vi "Double to RGB Image.vi"(8 "error in (no error)":errorcluster, 9 "minimum":sgl, 10 "maximum":sgl, 11 "Image Reference In":T1) -> (0 "error out":errorcluster, 3 "Image Reference Out":T1)   [LabVIEW 2019]
doc: "This VI converts a double image to a U8 image by converting the pixels from values in a particular range to 0-255 and adding them to a new image."
uses:
  <vilib>/vision/Image Controls.llb/IMAQ Image.ctl
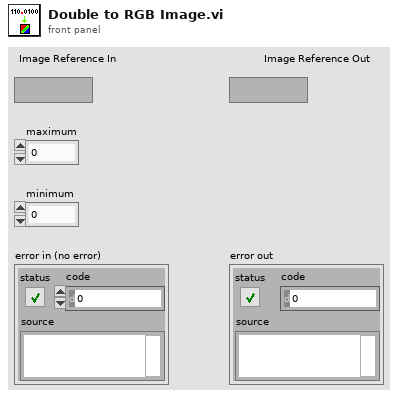
[diagram p1: front panel]
types:
  T1 = typedef "IMAQ Image.ctl" = refnum<image>
  T2 = typedef "Image Type" = u32
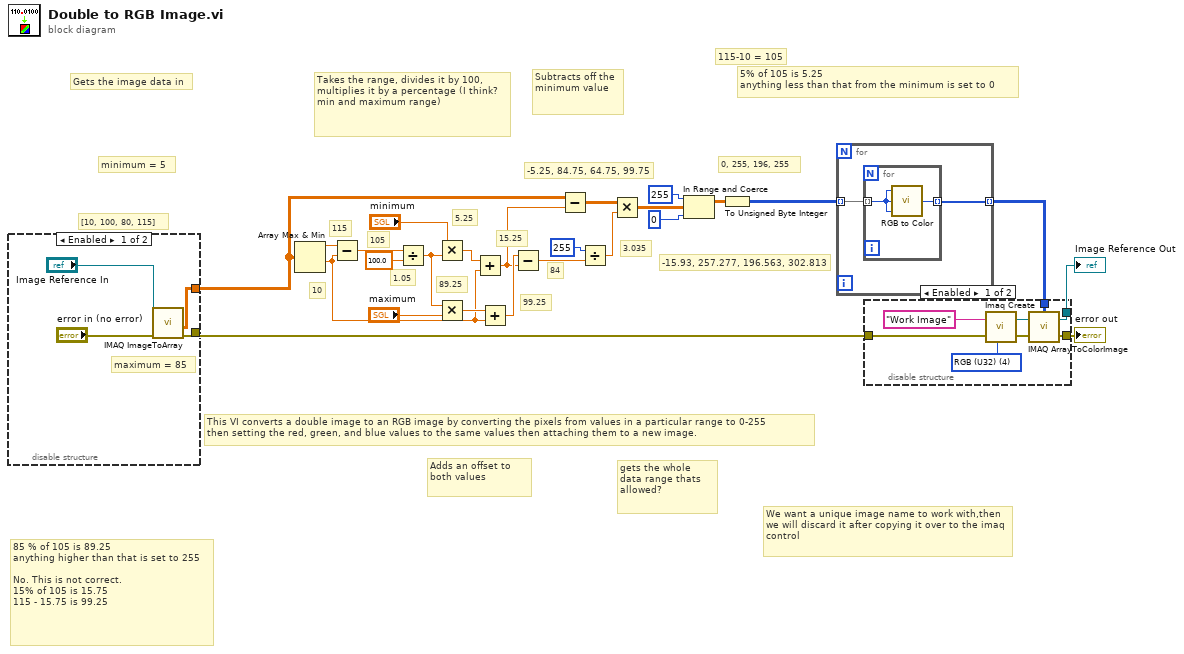
[diagram p0: block diagram]
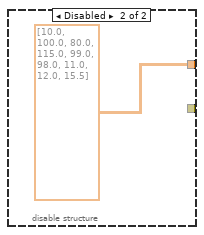
[diagram p3: hidden frame]
diagram:
  # "85 % of 105 is 89.25\nanything higher than that is set to 255\n\nNo. This is not correct.\n15% of 105 is 15.75\n115 - 15.75 is 99.25"
  # "5% of 105 is 5.25\nanything less than that from the minimum is set to 0"
  # "115-10 = 105"
  # "0, 255, 196, 255"
  # "-15.93, 257.277, 196.563, 302.813"
  # "-5.25, 84.75, 64.75, 99.75"
  # "3.035"
  # "84"
  # "99.25"
  # "15.25"
  # "89.25"
  # "5.25"
  # "maximum = 85"
  # "minimum = 5"
  # "1.05"
  # "105"
  # "10"
  # "115"
  # "[10, 100, 80, 115]"
  # "gets the whole data range thats allowed?"
  # "Subtracts off the minimum value"
  # "Adds an offset to both values"
  # "Takes the range, divides it by 100, multiplies it by a percentage (I think? min and maximum range)"
  # "Gets the image data in"
  # "We want a unique image name to work with,then we will discard it after copying it over to the imaq control"
  # "This VI converts a double image to an RGB image by converting the pixels from values in a particular range to 0-255\nthen setting the red, green, and blue values to the same values then attaching them to a new image."
  n1 = disable-structure shown="Enabled" {
    disable-tunnel: [w27 _] -> w20
    disable-tunnel: [w26 sgl[][] [[10.0], [100.0], [80.0], [115.0], [99.0], [98.0], [11.0], [12.0], [15.5]] ("Image Pixels (Float)")] -> w4
    frame Enabled {
      n2 = call "IMAQ ImageToArray"("error in (no error)"="error in (no error)", "Image"="Image Reference In") -> ("Image Pixels (Float)"=w26:sgl[][], "error out"=w27:errorcluster)  [unwired: 2 in, 3 out]
    }
    frame Disabled {
    }
  }
  n3 = Array Max & Min(array=w4) -> (max value=w22:sgl, min value=w9:sgl)  [unwired: 2 out]
  n4 = Subtract(x=w22, y=w9) -> (x-y=w16:sgl)
  n5 = Divide(x=w16, y=sgl 100.0) -> (x/y=w2:sgl)
  n6 = Multiply(x="minimum", y=w2) -> (x*y=w14:sgl)
  n7 = Multiply(x=w2, y="maximum") -> (x*y=w13:sgl)
  n8 = Add(x=w14, y=w9) -> (x+y=w10:sgl)
  n9 = Add(x=w13, y=w9) -> (x+y=w12:sgl)
  n10 = Subtract(x=w12, y=w10) -> (x-y=w11:sgl)
  n11 = Subtract(x=w4, y=w10) -> (x-y=w23:sgl[][])
  n12 = Divide(x=255, y=w11) -> (x/y=w25:sgl)
  n13 = Multiply(x=w23, y=w25) -> (x*y=w6:sgl[][])
  n14 = In Range and Coerce(upper limit=255, x=w6, lower limit=0) -> (coerced(x)=w5:sgl[][])  [unwired: 1 out]
  n15 = To Unsigned Byte Integer(number=w5) -> (unsigned 8bit integer=w21:u8[][])
  n16 = for {
    tunnel: w21 -> [w32] mode=indexing
    tunnel: [w31] -> w3 mode=indexing
    n17 = for {
      tunnel: w32 -> [w34] mode=indexing
      tunnel: [w33] -> w31 mode=indexing
      n18 = call <vilib>:"RGB to Color.vi"("B"=w34, "G"=w34, "R"=w34) -> ("Color"=w33:u32)
    }
  }
  n19 = disable-structure shown="Enabled" {
    disable-tunnel: w20 -> [w39 _]
    disable-tunnel: [w38 _] -> w19
    disable-tunnel: [w37 _] -> w18
    disable-tunnel: w3 -> [w36 _]
    frame Enabled {
      w42 = T2 4 items=["Grayscale (U8)", "Grayscale (I16)", "Grayscale (SGL)", "Complex (CSG)", "RGB (U32)", "HSL (U32)", "RGB (U64)", "Grayscale (U16)"] ("Image Type")
      n20 = call "Imaq Create"("Image Name"="Work Image", "Image Type"=w42, "error in (no error)"=w39) -> ("New Image"=w41:T1, "error out"=w40:errorcluster)  [unwired: 2 in]
      n21 = call "IMAQ ArrayToColorImage"("Image Pixels (U32)"=w36, "Image"=w41, "error in (no error)"=w40) -> ("Image Out"=w37:T1, "error out"=w38:errorcluster)  [unwired: 2 in]
    }
    frame Disabled {
    }
  }
  "error out" <- w19
  "Image Reference Out" <- w18
